vi "test_char limit case 2.vi"(8 "error in (no error)":errorcluster, 11 "TestCase in":refnum<class "Char Count Limit.lvclass">) -> (0 "error out":errorcluster, 3 "TestCase out":refnum<class "Char Count Limit.lvclass">)   [LabVIEW 2017, in "Char Count Limit.lvclass"]
uses:
  Char Count Limit.lvclass
  <vilib>/addons/_JKI Toolkits/VI Tester/TestCase.llb/TestCase.lvclass
  Libraries/SSH/SSH.lvlib
  C:/Program Files (x86)/National Instruments/LabVIEW 2017/vi.lib/addons/_JKI Toolkits/VI Tester/TestCase.llb/TestCase.lvclass
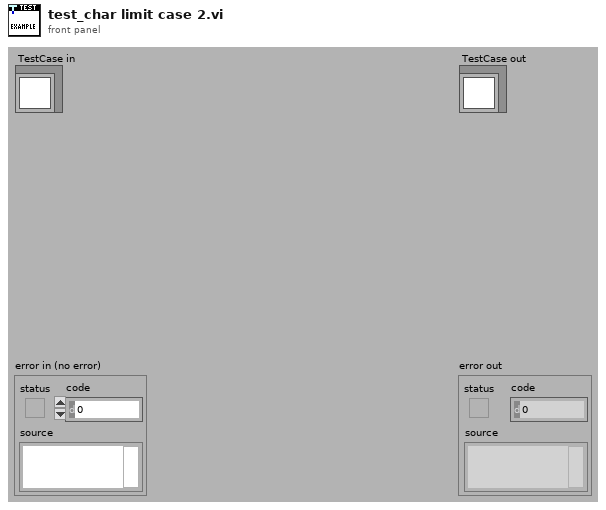
[diagram p1: front panel]
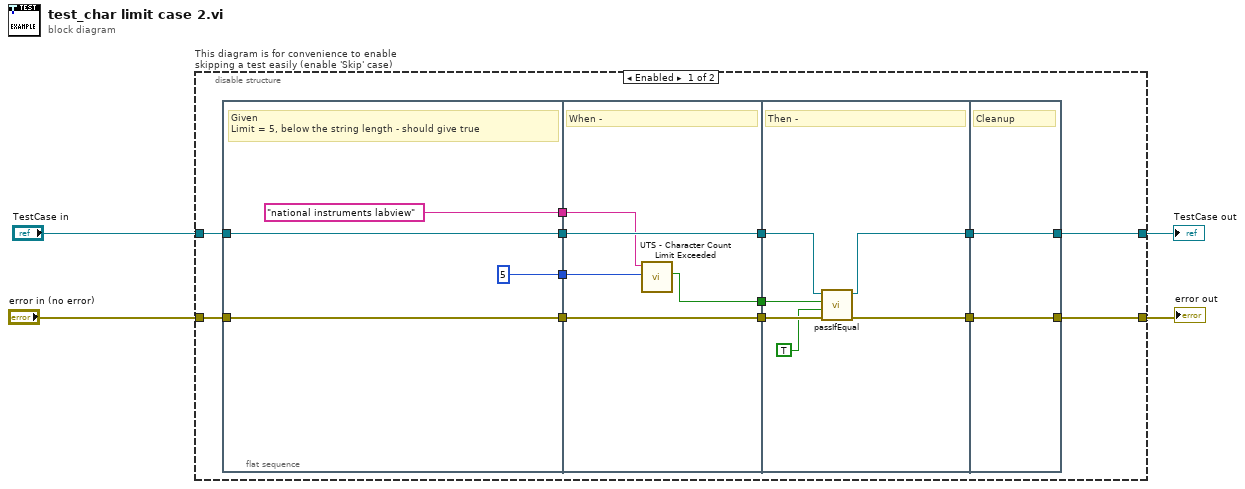
[diagram p0: block diagram]
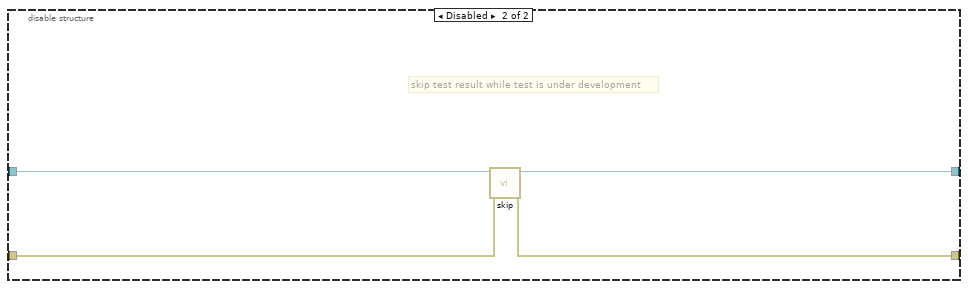
[diagram p2: hidden frame]
diagram:
  n1 = disable-structure "This diagram is for convenience to enable skipping a test easily (enable 'Skip' case)" shown="Enabled" {
    disable-tunnel: "TestCase in" -> [w11 w38]
    disable-tunnel: [w9 w36] -> w1
    disable-tunnel: [w8 w37] -> w3
    disable-tunnel: "error in (no error)" -> [w10 w35]
    frame Enabled {
      n2 = flat-sequence {
        tunnel: w10 -> [w20]
        tunnel: w11 -> [w21]
        tunnel: [w21] -> w17
        tunnel: [w20] -> w16
        tunnel: ["national instruments labview" ("Response String in")] -> w7
        tunnel: [5 ("Character Count Limit")] -> w6
        tunnel: [w26] -> w15
        tunnel: [w25] -> w14
        tunnel: w17 -> [w26]
        tunnel: w16 -> [w25]
        tunnel: w7 -> [w24]
        tunnel: w6 -> [w23]
        tunnel: [w22] -> w5
        tunnel: [w31] -> w13
        tunnel: [w29] -> w12
        tunnel: w15 -> [w32]
        tunnel: w14 -> [w30]
        tunnel: w5 -> [w28]
        tunnel: [w33] -> w8
        tunnel: [w34] -> w9
        tunnel: w13 -> [w34]
        tunnel: w12 -> [w33]
        frame #0 {
          # "Given\nLimit = 5, below the string length - should give true"
        }
        frame #1 {
          # "When -"
          n3 = call "UTS - Character Count Limit Exceeded.vi"("Character Count Limit"=w23, "Response String in"=w24) -> ("Limit Exceeded"=w22:bool)  [unwired: 9 in]
        }
        frame #2 {
          # "Then -"
          n4 = call-dynamic "passIfEqual.vi"("error in (no error)"=w30, "y"=TRUE, "x"=w28, "TestCase in"=w32) -> ("error out"=w29:errorcluster, "TestCase out"=w31:refnum<class "Char Count Limit.lvclass">)  [unwired: 6 in]
        }
        frame #3 {
          # "Cleanup"
        }
      }
    }
    frame Disabled {
      # "skip test result while test is under development"
      n5 = call <vilib>:"skip.vi"("error in (no error)"=w35, "TestCase in"=w38) -> ("error out"=w37:errorcluster, "TestCase out"=w36:refnum<class "Char Count Limit.lvclass">)  [unwired: 8 in]
    }
  }
  "error out" <- w3
  "TestCase out" <- w1
